vi "select_initial_historian_1tuple.vi"(9 "time":timestamp, 10 "Column table":string[](array[string]), 11 "table":string) -> (3 "parameters":string)   [LabVIEW 2019, in "PostgreSQL.lvlib"]
uses:
  PostgreSQL.lvlib
panel:
  out "Data to write":bool
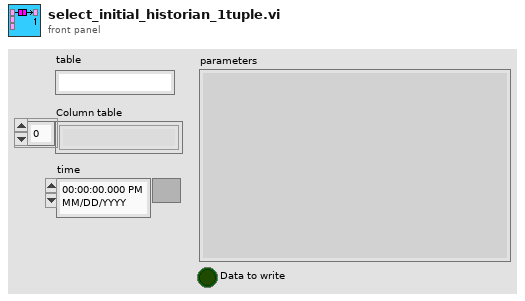
[diagram p1: front panel]
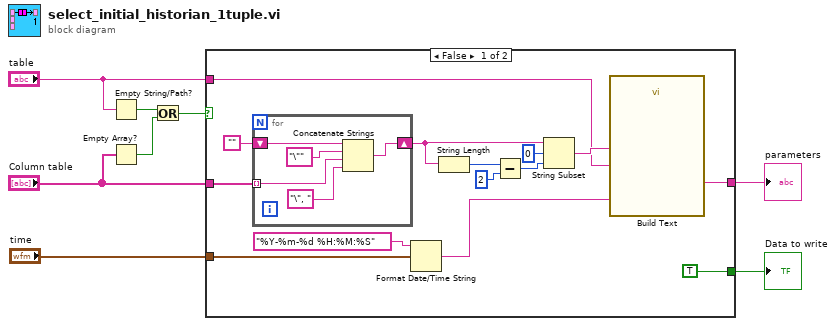
[diagram p0: block diagram]
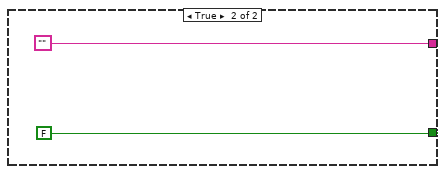
[diagram p2: hidden frame]
diagram:
  n1 = Empty String/Path?(string/path="table") -> (empty?=w5:bool)
  n2 = Empty Array?(array="Column table") -> (empty?=w4:bool)
  n3 = Or(x=w5, y=w4) -> (x .or. y?=w3:bool)
  n4 = case shown="False" w3 {
    tunnel: [w12 ""] -> w8
    tunnel: "table" -> [w13 _]
    tunnel: "Column table" -> [w16 _]
    tunnel: [TRUE FALSE] -> w2
    tunnel: "time" -> [w9 _]
    frame False {
      n5 = for {
        shift-right: [w25] -> w22
        shift-left: "" -> [w23]
        tunnel: w16 -> [w24] mode=indexing
        n6 = Concatenate Strings(w23, "\"" ("table"), w24, "\", " ("table")) -> (w25:string)
      }
      n7 = Format Date/Time String(time format string (%c)="%Y-%m-%d %H:%M:%S", seconds (now)=w9) -> (date/time string=w10:string)  [unwired: 1 in]
      n8 = String Length(string=w22) -> (length=w21:i32)
      n9 = Subtract(x=w21, y=2) -> (x-y=w19:i32)
      n10 = String Subset(string=w22, offset (0)=0, length (rest)=w19) -> (substring=w14:string)
      n11 = call "Build Text"("columns"=w14, "table"=w13, "time"=w10) -> ("Result"=w12:string)  [unwired: 11 in, 1 out]
    }
    frame True {
    }
  }
  "parameters" <- w8
  "Data to write" <- w2
